vi "Peak-List-Test.vi"() -> ()   [LabVIEW 2014]
uses:
  <vilib>/Analysis/2dsp.llb/Integral Method.ctl
  <vilib>/Analysis/8numeric.llb/1D Numeric Integration.vi
  <vilib>/Analysis/NI_AALPro.lvlib
  <vilib>/Analysis/NI_AAL_SigProc.lvlib
panel:
  out "delta WL":dbl=0.7806262402999664
  out "appended array":string[][](array[string])=[["28865", "1036", "109300", "1961"], ["28453", "1024", "108350", "1940"]]
  in  "threshold":dbl=200.0 format="%0.2f"
  out "table":string[][](table)=[["Name", "Integration", "Peak"], ["Laser", "28453", "1024"], ["Laser2", "108350", "1940"]]
  out "Waveform Graph":dbl[][](graph)=[[3.587878787878765, 3.587878787878765, 5.587878787878765, 4.587878787878765, 17.587878787878765, 6.587878787878765, 7.587878787878765, 3.587878787878765, 4.587878787878765, 4.587878787878765, 4.587878787878765, 10.587878787878765, 7.587878787878765, 5.587878787878765, 7.587878787878765, 3.587878787878765, 4.587878787878765, 2.587878787878765, 8.587878787878765, 6.587878787878765, 5.587878787878765, 11.587878787878765, 5.587878787878765, 9.587878787878765, 15.587878787878765, 3.587878787878765, 8.587878787878765, 11.587878787878765, 8.587878787878765, 16.587878787878765, 15.587878787878765, 19.587878787878765, 15.587878787878765, 13.587878787878765, 28.587878787878765, 26.587878787878765, 27.587878787878765, 37.587878787878765, 31.587878787878765, 42.587878787878765, 52.587878787878765, 45.587878787878765, 65.58787878787876, 73.58787878787876, 75.58787878787876, 98.58787878787876, 95.58787878787876, 121.58787878787876, 126.58787878787876, 148.58787878787876, 153.58787878787876, 166.58787878787876, 188.58787878787876, 206.58787878787876, 231.58787878787876, 250.58787878787876, 276.58787878787876, 294.58787878787876, 335.58787878787876, 364.58787878787876, 399.58787878787876, 426.58787878787876, 473.58787878787876, 534.5878787878787, 566.5878787878787, 615.5878787878787, 658.5878787878787, 705.5878787878787, 746.5878787878787, 751.5878787878787, 870.5878787878787, 854.5878787878787, 917.5878787878787, 981.5878787878787, 1002.5878787878787, 994.5878787878787, 1043.5878787878787, 1041.5878787878787, 989.5878787878787, 989.5878787878787, 1003.5878787878787, 981.5878787878787, 901.5878787878787, 886.5878787878787, 854.5878787878787, 794.5878787878787, 757.5878787878787, 696.5878787878787, 652.5878787878787, 622.5878787878787, 553.5878787878787, 526.5878787878787, 514.5878787878787, 452.58787878787876, 420.58787878787876, 392.58787878787876, 355.58787878787876, 340.58787878787876, 329.58787878787876, 295.58787878787876, 284.58787878787876, 259.58787878787876, 236.58787878787876, 238.58787878787876, 217.58787878787876, 199.58787878787876, 180.58787878787876, 177.58787878787876, 162.58787878787876, 151.58787878787876, 145.58787878787876, 135.58787878787876, 119.58787878787876, 115.58787878787876, 104.58787878787876, 95.58787878787876, 89.58787878787876, 80.58787878787876, 78.58787878787876, 71.58787878787876, 72.58787878787876, 66.58787878787876, 55.587878787878765, 58.587878787878765, 55.587878787878765, 51.587878787878765, 46.587878787878765, 50.587878787878765, 39.587878787878765, 40.587878787878765, 34.587878787878765, 39.587878787878765, 30.587878787878765, 28.587878787878765, 25.587878787878765, 33.587878787878765, 30.587878787878765, 27.587878787878765, 27.587878787878765, 25.587878787878765, 28.587878787878765, 22.587878787878765, 24.587878787878765, 25.587878787878765, 16.587878787878765, 12.587878787878765, 22.587878787878765, 14.587878787878765, 25.587878787878765, 22.587878787878765, 15.587878787878765, 16.587878787878765, 19.587878787878765, 18.587878787878765, 17.587878787878765, 7.587878787878765, 17.587878787878765, 18.587878787878765, 17.587878787878765, 16.587878787878765, 17.587878787878765, 15.587878787878765, 14.587878787878765, 15.587878787878765, 11.587878787878765, 9.587878787878765, 12.587878787878765, 10.587878787878765, 15.587878787878765, 19.587878787878765, 17.587878787878765, 20.587878787878765, 15.587878787878765, 15.587878787878765, 14.587878787878765, 13.587878787878765, 12.587878787878765, 13.587878787878765, 11.587878787878765, 12.587878787878765, 14.587878787878765, 15.587878787878765, 18.587878787878765, 0.0, 0.0, 0.0, 0.0, 0.0, 0.0, 0.0, 0.0, 0.0, 0.0, 0.0, 0.0, 0.0, 0.0, 0.0, 0.0, 0.0, 0.0, 0.0, 0.0, 0.0, 0.0, 0.0, 0.0, 0.0, 0.0, 0.0, 0.0, 0.0, 0.0, 0.0, 0.0, 0.0, 0.0, 0.0, 0.0, 0.0, 0.0, 0.0, 0.0, 0.0, 0.0, 0.0, 0.0, 0.0, 0.0, 0.0, 0.0, 0.0, 0.0, 0.0, 0.0, 0.0, 0.0, 0.0, 0.0, 0.0, 0.0, 0.0, 0.0, 0.0, 0.0, 0.0, 0.0, 0.0, 0.0, 0.0, 0.0, 0.0, 0.0, 0.0, 0.0, 0.0, 0.0, 0.0, 0.0, 0.0, 0.0, 0.0, 0.0, 0.0, 0.0, 0.0, 0.0, 0.0, 0.0, 0.0, 0.0], [174.58787878787876, 192.58787878787876, 212.58787878787876, 247.58787878787876, 262.58787878787876, 307.58787878787876, 346.58787878787876, 383.58787878787876, 427.58787878787876, 491.58787878787876, 546.5878787878787, 599.5878787878787, 661.5878787878787, 737.5878787878787, 803.5878787878787, 892.5878787878787, 971.5878787878787, 1051.5878787878787, 1155.5878787878787, 1247.5878787878787, 1306.5878787878787, 1360.5878787878787, 1464.5878787878787, 1555.5878787878787, 1598.5878787878787, 1640.5878787878787, 1722.5878787878787, 1753.5878787878787, 1805.5878787878787, 1806.5878787878787, 1867.5878787878787, 1888.5878787878787, 1925.5878787878787, 1940.5878787878787, 1922.5878787878787, 1936.5878787878787, 1929.5878787878787, 1930.5878787878787, 1940.5878787878787, 1920.5878787878787, 1887.5878787878787, 1866.5878787878787, 1843.5878787878787, 1862.5878787878787, 1842.5878787878787, 1796.5878787878787, 1778.5878787878787, 1743.5878787878787, 1716.5878787878787, 1680.5878787878787, 1687.5878787878787, 1645.5878787878787, 1613.5878787878787, 1582.5878787878787, 1571.5878787878787, 1539.5878787878787, 1536.5878787878787, 1490.5878787878787, 1465.5878787878787, 1419.5878787878787, 1410.5878787878787, 1396.5878787878787, 1370.5878787878787, 1345.5878787878787, 1329.5878787878787, 1295.5878787878787, 1276.5878787878787, 1230.5878787878787, 1210.5878787878787, 1200.5878787878787, 1191.5878787878787, 1157.5878787878787, 1114.5878787878787, 1097.5878787878787, 1081.5878787878787, 1062.5878787878787, 1036.5878787878787, 1001.5878787878787, 983.5878787878787, 941.5878787878787, 936.5878787878787, 908.5878787878787, 903.5878787878787, 874.5878787878787, 862.5878787878787, 818.5878787878787, 809.5878787878787, 786.5878787878787, 751.5878787878787, 738.5878787878787, 717.5878787878787, 684.5878787878787, 690.5878787878787, 662.5878787878787, 635.5878787878787, 631.5878787878787, 600.5878787878787, 576.5878787878787, 563.5878787878787, 549.5878787878787, 538.5878787878787, 531.5878787878787, 502.58787878787876, 495.58787878787876, 475.58787878787876, 469.58787878787876, 454.58787878787876, 448.58787878787876, 426.58787878787876, 422.58787878787876, 409.58787878787876, 397.58787878787876, 377.58787878787876, 371.58787878787876, 360.58787878787876, 356.58787878787876, 345.58787878787876, 338.58787878787876, 324.58787878787876, 313.58787878787876, 303.58787878787876, 290.58787878787876, 292.58787878787876, 285.58787878787876, 273.58787878787876, 269.58787878787876, 251.58787878787876, 252.58787878787876, 247.58787878787876, 241.58787878787876, 228.58787878787876, 217.58787878787876, 217.58787878787876, 217.58787878787876, 209.58787878787876, 195.58787878787876, 199.58787878787876, 192.58787878787876, 185.58787878787876, 185.58787878787876, 180.58787878787876, 176.58787878787876, 176.58787878787876, 174.58787878787876, 163.58787878787876, 158.58787878787876, 151.58787878787876, 155.58787878787876, 149.58787878787876, 145.58787878787876, 137.58787878787876, 132.58787878787876, 123.58787878787876, 135.58787878787876, 129.58787878787876, 123.58787878787876, 116.58787878787876, 123.58787878787876, 117.58787878787876, 101.58787878787876, 105.58787878787876, 99.58787878787876, 98.58787878787876, 99.58787878787876, 95.58787878787876, 86.58787878787876, 97.58787878787876, 92.58787878787876, 85.58787878787876, 77.58787878787876, 79.58787878787876, 78.58787878787876, 79.58787878787876, 84.58787878787876, 75.58787878787876, 77.58787878787876, 70.58787878787876, 62.587878787878765, 71.58787878787876, 63.587878787878765, 60.587878787878765, 60.587878787878765, 55.587878787878765, 54.587878787878765, 52.587878787878765, 62.587878787878765, 51.587878787878765, 49.587878787878765, 43.587878787878765, 55.587878787878765, 50.587878787878765, 40.587878787878765, 44.587878787878765, 46.587878787878765, 46.587878787878765, 40.587878787878765, 38.587878787878765, 42.587878787878765, 36.587878787878765, 36.587878787878765, 39.587878787878765, 38.587878787878765, 29.587878787878765, 30.587878787878765, 30.587878787878765, 31.587878787878765, 32.587878787878765, 31.587878787878765, 30.587878787878765, 31.587878787878765, 27.587878787878765, 25.587878787878765, 31.587878787878765, 22.587878787878765, 23.587878787878765, 28.587878787878765, 22.587878787878765, 21.587878787878765, 18.587878787878765, 23.587878787878765, 52.587878787878765, 29.587878787878765, 22.587878787878765, 20.587878787878765, 13.587878787878765, 16.587878787878765, 18.587878787878765, 23.587878787878765, 17.587878787878765, 15.587878787878765, 17.587878787878765, 24.587878787878765, 13.587878787878765, 11.587878787878765, 18.587878787878765, 16.587878787878765, 11.587878787878765, 16.587878787878765, 10.587878787878765, 18.587878787878765, 16.587878787878765, 11.587878787878765, 13.587878787878765, 15.587878787878765, 8.587878787878765, 9.587878787878765, 12.587878787878765, 9.587878787878765, 10.587878787878765, 10.587878787878765, 11.587878787878765, 13.587878787878765, 17.587878787878765, 10.587878787878765, 9.587878787878765, 13.587878787878765, 13.587878787878765, 9.587878787878765, 8.587878787878765, 4.587878787878765, 8.587878787878765, 8.587878787878765, 5.587878787878765, 7.587878787878765, 8.587878787878765, 7.587878787878765, 16.587878787878765, 12.587878787878765, 5.587878787878765, 10.587878787878765, 11.587878787878765]]
  out "XY Graph":T1(graph)
  in  "Range List":T2(array[cluster])=[{"Name"="Laser", "Inicial"=400.0, "Final"=540.0}, {"Name"="Laser2", "Inicial"=600.0, "Final"=800.0}]
  in  "Select Light Source":u16(ring)=6
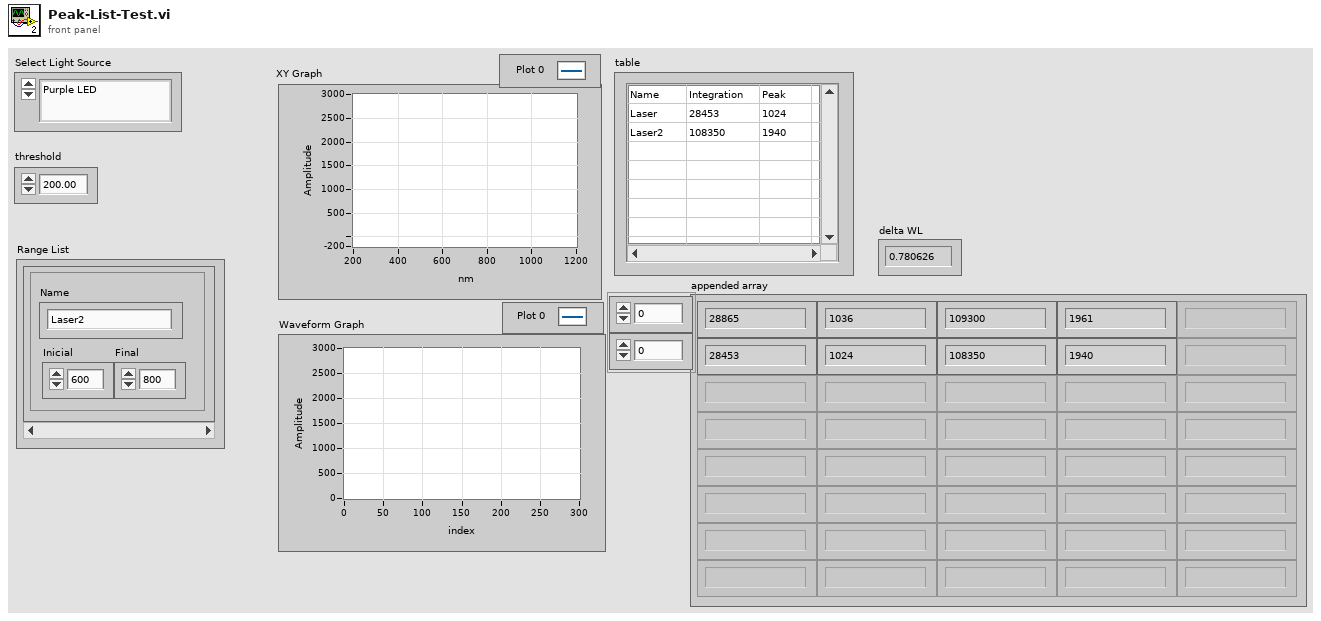
[diagram p1: front panel]
types:
  T1 = cluster{"WL Values":dbl[], "Spectrum Values":dbl[]}
  T2 = cluster{"Name":string, "Inicial":dbl, "Final":dbl}[]
  T3 = typedef "NI_AALPro.lvlib/Integral Method.ctl" = i32
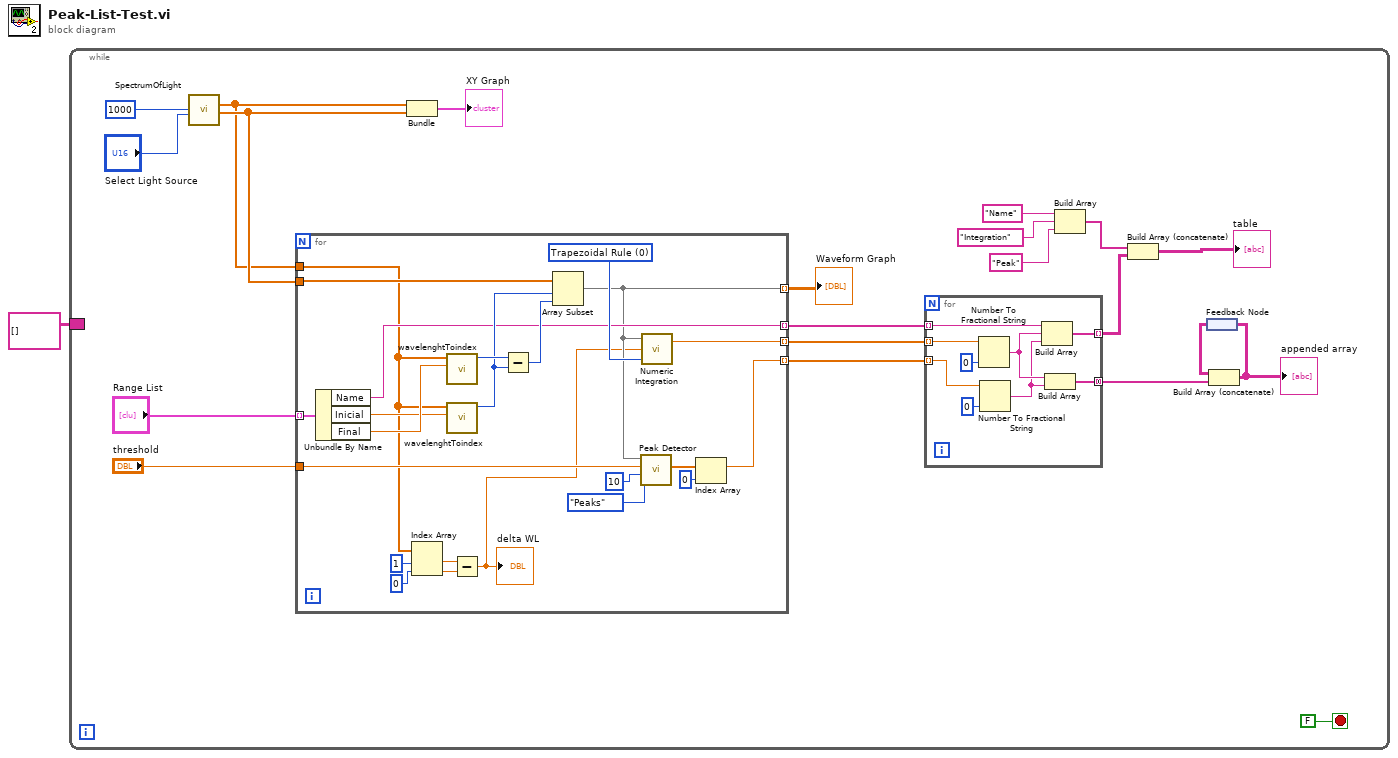
[diagram p0: block diagram]
diagram:
  n1 = while {
    border: string[][] [] -> [_]
    stop <- FALSE stop-if-true
    n2 = call "SpectrumOfLight.vi"("Select Light Source"="Select Light Source", "Integration Time (ms)"=u32 1000) -> ("Spectrum Values"=w19:dbl[], "WL Values"=w2:dbl[])  [unwired: 8 in]
    n3 = for {
      tunnel: w2 -> [w33]
      tunnel: w19 -> [w51]
      tunnel: "Range List" -> [w54] mode=indexing
      tunnel: [w44] -> w17 mode=indexing
      tunnel: [w46] -> w12 mode=indexing
      tunnel: [w45] -> w11 mode=indexing
      tunnel: "threshold" -> [w43]
      tunnel: [w39] -> w8 mode=indexing
      w47 = T3 0 items=["Trapezoidal Rule", "Simpson's Rule", "Simpson's 3/8 Rule", "Bode Rule"] ("integration method")
      n4 = Unbundle By Name(w54) -> ("Name"=w45:string, "Inicial"=w52:dbl, "Final"=w53:dbl)
      n5 = Index Array(array=w33, index #1=1 ("index"), index #2=0 ("index")) -> (element #1=w34:dbl, element #2=w35:dbl)
      n6 = call "wavelenghtToindex.vi"("WL in"=w53, "WL Values"=w33) -> ("index of WL"=w50:i32)  [unwired: 9 in]
      n7 = call "wavelenghtToindex.vi"("WL in"=w52, "WL Values"=w33) -> ("index of WL"=w48:i32)  [unwired: 9 in]
      n8 = Subtract(x=w34, y=w35) -> (x-y=w32:dbl)
      "delta WL" <- w32
      n9 = Subtract(x=w50, y=w48) -> (x-y=w49:i32)
      n10 = Array Subset(array=w51, index=w48, length=w49) -> (w44:dbl[])
      n11 = call <vilib>:"Peak Detector.vi"("peaks/valleys"=enum32{"Peaks", "Valleys"}."Peaks", "width"=10, "threshold"=w43, "X"=w44) -> ("Amplitudes"=w40:dbl[])  [unwired: 3 in, 4 out]
      n12 = call-poly <vilib>:"Numeric Integration.vi"("integration method"=w47, "dt"=w32, "Input Array"=w44) -> ("result"=w46:dbl)  [unwired: 1 out]
      n13 = Index Array(array=w40, index=0) -> (element=w39:dbl)
    }
    "Waveform Graph" <- w17
    n14 = Bundle("WL Values"=w2, "Spectrum Values"=w19) -> (→"XY Graph":T1)  [unwired: 1 in]
    n15 = for {
      tunnel: w12 -> [w31] mode=indexing
      tunnel: w11 -> [w29] mode=indexing
      tunnel: [w28] -> w10 mode=indexing
      tunnel: w8 -> [w26] mode=indexing
      tunnel: [w23] -> w4 mode=concatenating
      n16 = Number To Fractional String(number=w31, precision (6)=i16 0) -> (F-format string=w25:string)  [unwired: 2 in]
      n17 = Number To Fractional String(number=w26, precision (6)=i16 0) -> (F-format string=w24:string)  [unwired: 2 in]
      n18 = Build Array(w29, w25, w24) -> (w28:string[])
      n19 = Build Array(w25, w24) -> (w23:string[])
    }
    n20 = Build Array("Name", "Integration", "Peak") -> (w16:string[])
    n21 = Build Array (concatenate)(w16, w10) -> (→"table":string[][])
    n22 = feedback #1() -> (w5:string[][])
    n23 = Build Array (concatenate)(w5, w4) -> (w6:string[][])
    "appended array" <- w6
    n24 = feedback-in #1(w6) -> ()
  }
